vi "Launcher.vi"   [LabVIEW 2018]
uses:
  Chat Room/Chat Room/Chat Room.lvclass
  C:/Program Files (x86)/National Instruments/LabVIEW 2018/vi.lib/ActorFramework/Actor/Actor.lvclass
  <vilib>/ActorFramework/Stop Msg/Stop Msg.lvclass/Stop Msg.ctl
  <vilib>/ActorFramework/Message Enqueuer/Message Enqueuer.lvclass/Message Enqueuer.ctl
  <vilib>/ActorFramework/Message Enqueuer/Enqueue Critical.vi
  <vilib>/ActorFramework/Stop Msg/Stop Msg.lvclass
  C:/Program Files (x86)/National Instruments/LabVIEW 2018/vi.lib/ActorFramework/Message/Message.lvclass
  <vilib>/ActorFramework/Message Priority Queue/Priority Enqueue.vi
  <vilib>/ActorFramework/Actor/Actor.lvclass
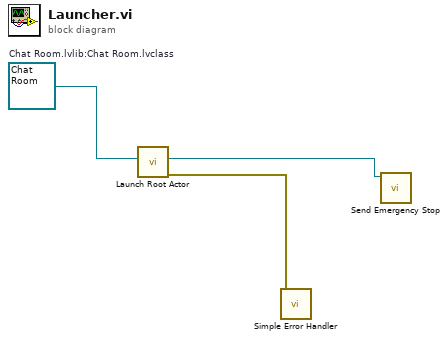
[diagram p0: block diagram]
diagram:
  w3 = refnum<class "Chat Room.lvclass"> refnum  # Chat Room.lvlib:Chat Room.lvclass
  n1 = call <vilib>:"Launch Root Actor.vi"("Actor"=w3) -> ("error out"=w2:errorcluster, "Actor's Enqueuer"=w1:refnum<class "Message Enqueuer.lvclass">)  [unwired: 9 in]
  n2 = call <vilib>:"Simple Error Handler.vi"("error in (no error)"=w2) -> ()  [unwired: 4 in, 5 out]
  n3 = call <vilib>:"Send Emergency Stop.vi"("Message Enqueuer"=w1) -> ()  [unwired: 10 in, 1 out]
